vi "Display Lab Panel V4.83.vi"() -> ()   [LabVIEW 2012]
uses:
  Global display 1.vi
  Global display 2.vi
panel:
  in  "Tab Control 2":T1(tab)
  out "SIG LAB05-2":T2 {"PF" format="%.2f"; "AMPS" format="%.1f"}
  out "SIG LAB05-1":T2 {"PF" format="%.2f"; "AMPS" format="%.1f"}
  out "SIG LAB04-2":T2 {"PF" format="%.2f"; "AMPS" format="%.1f"}
  out "SIG LAB04-1":T2 {"PF" format="%.2f"; "AMPS" format="%.1f"}
  out "SIG LAB03-2":T2 {"PF" format="%.2f"; "AMPS" format="%.1f"}
  out "SIG LAB03-1":T2 {"PF" format="%.2f"; "AMPS" format="%.1f"}
  out "SIG LAB02-2":T2 {"PF" format="%.2f"; "AMPS" format="%.1f"}
  in  "RUN LAB01-1":bool
  in  "O/I  LAB05-1":bool
  in  "O/I  LAB05-2":bool
  in  "O/I  LAB04-1":bool
  in  "O/I  LAB04-2":bool
  in  "O/I  LAB02-1":bool
  in  "O/I  LAB02-2":bool
  in  "O/I  LAB01-2":bool
  in  "O/I  LAB01-1":bool
  in  "O/I  LAB03-1":bool
  in  "RUN LAB05-2":bool
  in  "RUN LAB05-1":bool
  in  "RUN LAB04-2":bool
  in  "RUN LAB04-1":bool
  in  "RUN LAB03-2":bool
  in  "RUN LAB03-1":bool
  in  "RUN LAB02-2":bool
  in  "RUN LAB02-1":bool
  in  "RUN LAB01-2":bool
  in  "SELECT LAB05-2":T3(radio)
  in  "SELECT LAB05-1":T3(radio)
  in  "SELECT LAB04-2":T3(radio)
  in  "SELECT LAB04-1":T3(radio)
  in  "SELECT LAB03-2":T3(radio)
  in  "SELECT LAB03-1":T3(radio)
  in  "SELECT LAB02-2":T3(radio)
  in  "SELECT LAB02-1":T3(radio)
  in  "SELECT LAB01-2":T3(radio)
  in  "SELECT LAB01-1":T3(radio)
  in  "O/I  LAB03-2":bool
  out "SIG LAB01-1":T2 {"PF" format="%.2f"; "AMPS" format="%.1f"}
  out "SIG LAB01-2":T2 {"PF" format="%.2f"; "AMPS" format="%.1f"}
  out "SIG LAB02-1":T2 {"PF" format="%.2f"; "AMPS" format="%.1f"}
  out "DISP LAB05-2":T4 {"MINS" format="%.2g"}
  out "DISP LAB05-1":T4 {"MINS" format="%.2g"}
  out "DISP LAB04-2":T4 {"MINS" format="%.2g"}
  out "DISP LAB04-1":T4 {"MINS" format="%.2g"}
  out "DISP LAB03-2":T4 {"MINS" format="%.2g"}
  out "DISP LAB03-1":T4 {"MINS" format="%.2g"}
  in  "SET LAB05-2":T5={"NAME"="", "DESCRIPTION"="", "CYCLES"=5.0, "T-RISE mins"=0.0, "T-RISE deg C"=0.0} {"CYCLES" min=5.0 step=1.0}
  in  "SET LAB05-1":T5={"NAME"="", "DESCRIPTION"="", "CYCLES"=5.0, "T-RISE mins"=0.0, "T-RISE deg C"=0.0} {"CYCLES" min=5.0 step=1.0}
  in  "SET LAB04-2":T5={"NAME"="", "DESCRIPTION"="", "CYCLES"=5.0, "T-RISE mins"=0.0, "T-RISE deg C"=0.0} {"CYCLES" min=5.0 step=1.0}
  in  "SET LAB04-1":T5={"NAME"="", "DESCRIPTION"="", "CYCLES"=5.0, "T-RISE mins"=0.0, "T-RISE deg C"=0.0} {"CYCLES" min=5.0 step=1.0}
  in  "SET LAB03-2":T5={"NAME"="", "DESCRIPTION"="", "CYCLES"=5.0, "T-RISE mins"=0.0, "T-RISE deg C"=0.0} {"CYCLES" min=5.0 step=1.0}
  in  "SET LAB03-1":T5={"NAME"="", "DESCRIPTION"="", "CYCLES"=5.0, "T-RISE mins"=0.0, "T-RISE deg C"=0.0} {"CYCLES" min=5.0 step=1.0}
  out "DISP LAB02-2":T4 {"MINS" format="%.2g"}
  out "DISP LAB02-1":T4 {"MINS" format="%.2g"}
  in  "SET LAB02-2":T5={"NAME"="", "DESCRIPTION"="", "CYCLES"=5.0, "T-RISE mins"=0.0, "T-RISE deg C"=0.0} {"CYCLES" min=5.0 step=1.0}
  in  "SET LAB02-1":T5={"NAME"="", "DESCRIPTION"="", "CYCLES"=5.0, "T-RISE mins"=0.0, "T-RISE deg C"=0.0} {"CYCLES" min=5.0 step=1.0}
  out "RESULT LAB05-2":bool
  out "RESULT LAB05-1":bool
  out "RESULT LAB04-2":bool
  out "RESULT LAB04-1":bool
  out "RESULT LAB03-2":bool
  out "RESULT LAB03-1":bool
  out "RESULT LAB02-2":bool
  out "RESULT LAB02-1":bool
  out "RESULT LAB01-2":bool
  out "RESULT LAB01-1":bool
  in  "SET LAB01-1":T5={"NAME"="", "DESCRIPTION"="", "CYCLES"=5.0, "T-RISE mins"=0.0, "T-RISE deg C"=0.0} {"CYCLES" min=5.0 step=1.0}
  in  "SET LAB01-2":T5={"NAME"="", "DESCRIPTION"="", "CYCLES"=5.0, "T-RISE mins"=0.0, "T-RISE deg C"=0.0} {"CYCLES" min=5.0 step=1.0}
  out "DISP LAB01-1":T4 {"MINS" format="%.2g"}
  out "DISP LAB01-2":T4 {"MINS" format="%.2f"}
  out "TEST VOLTS CHART":dynamicdata(graph)
  out "TEST AMPS CHART":dynamicdata(graph)
  out "TEMPERATURE (N) CHART":dynamicdata(graph)
  out "TEMPERATURE (L) CHART":dynamicdata(graph)
  # "LAB01"
  # "LAB02"
  # "LAB05"
  # "LAB03"
  # "LAB04"
  # "LAB01"
  # "LAB02"
  # "LAB03"
  # "LAB04"
  # "LAB05"
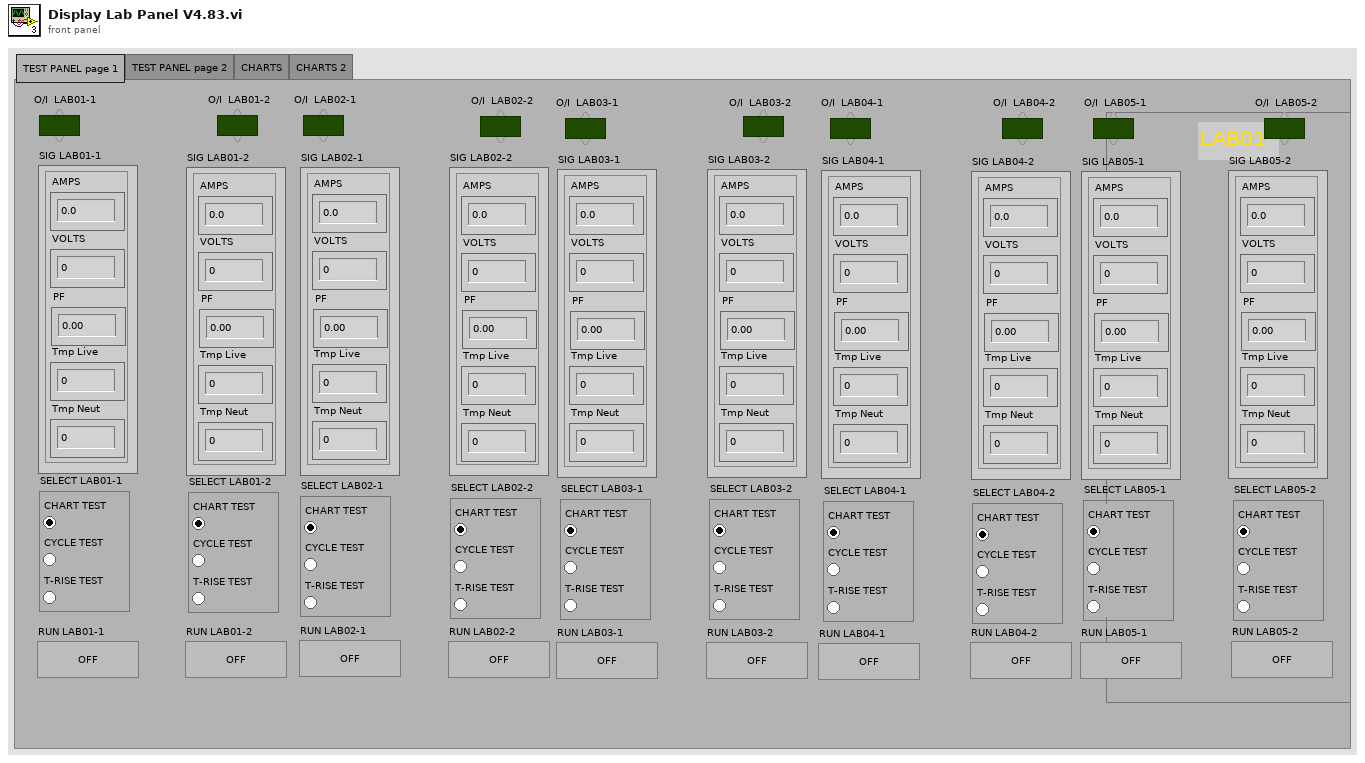
[diagram p1: front panel]
types:
  T1 = enum32{"TEST PANEL page 1", "TEST PANEL page 2", "CHARTS", "CHARTS 2"}
  T2 = cluster{"AMPS":dbl, "VOLTS":dbl, "PF":dbl, "Tmp Live":dbl, "Tmp Neut":dbl}
  T3 = enum32{"CHART TEST", "CYCLE TEST", "T-RISE TEST"}
  T4 = cluster{"CYCLE":dbl, "MINS":dbl, "STATUS":string}
  T5 = cluster{"NAME":string, "DESCRIPTION":string, "CYCLES":dbl, "T-RISE mins":dbl, "T-RISE deg C":dbl}
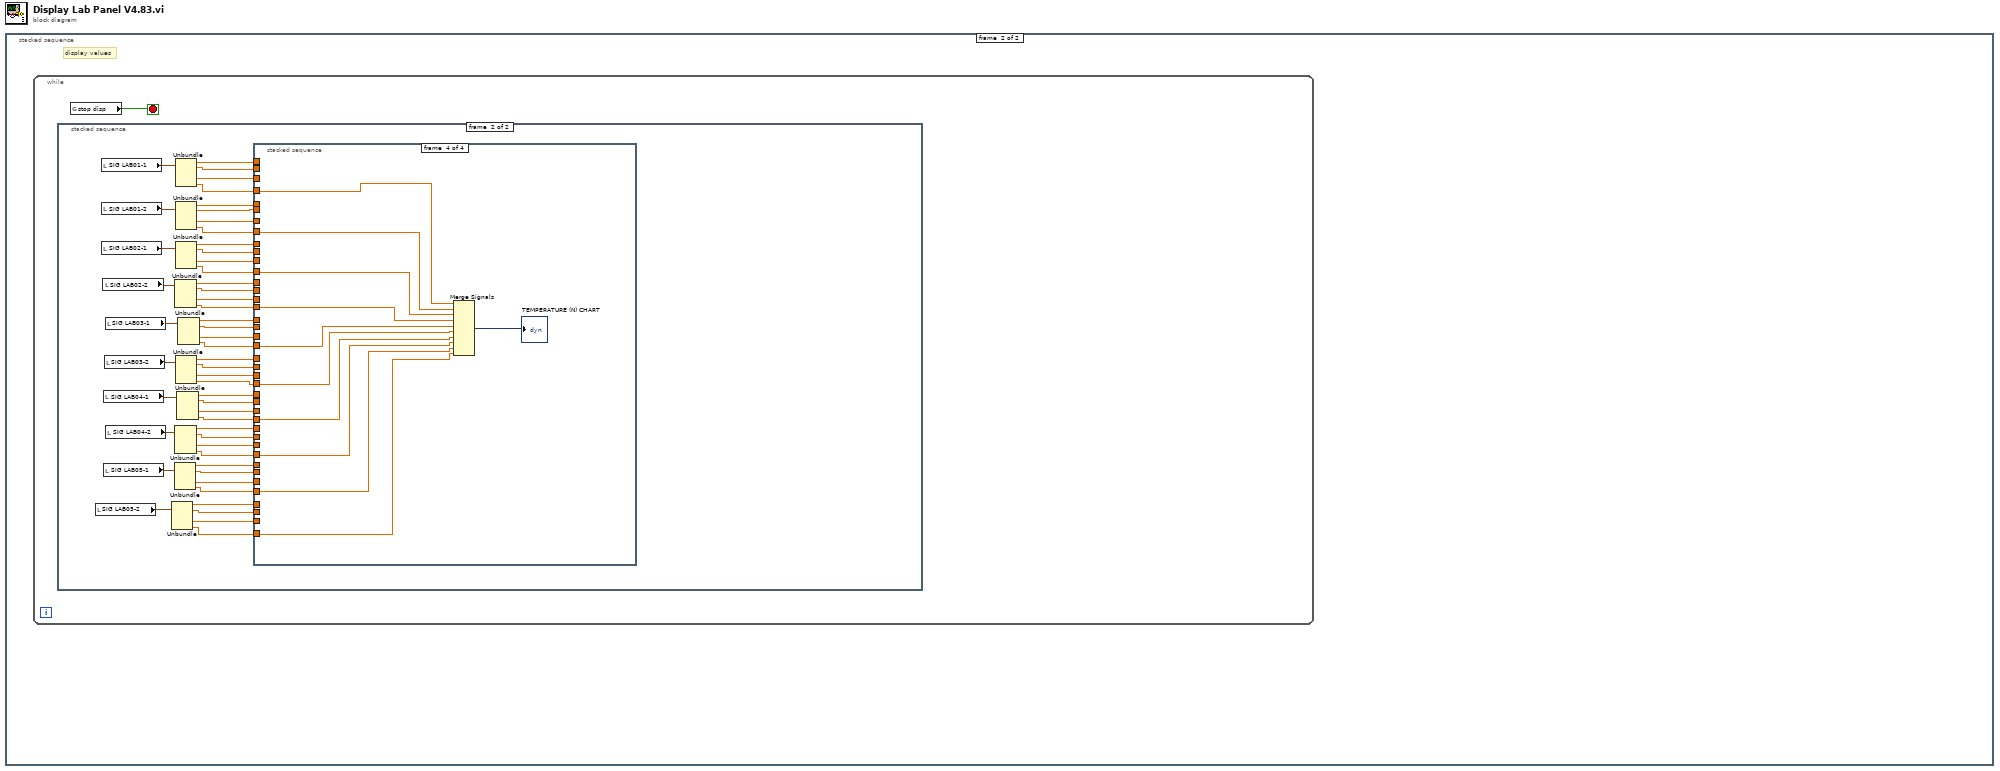
[diagram p0: block diagram]
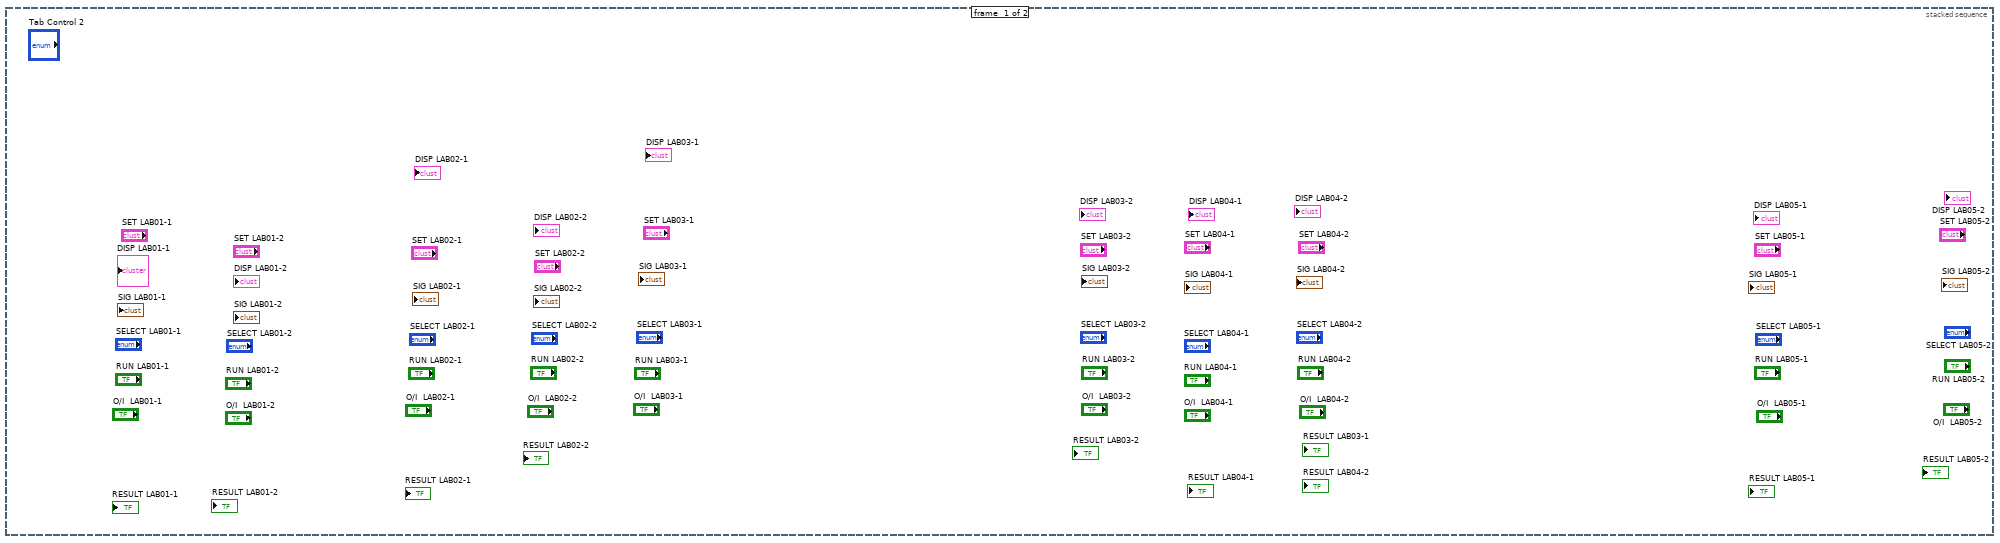
[diagram p2: hidden frame]
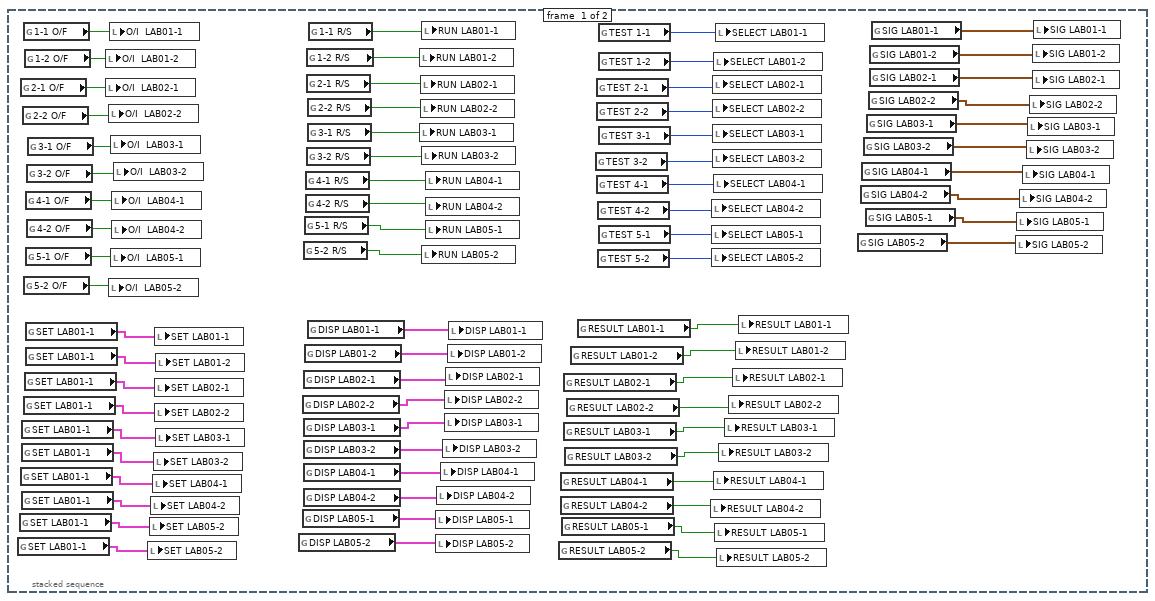
[diagram p3: hidden frame]
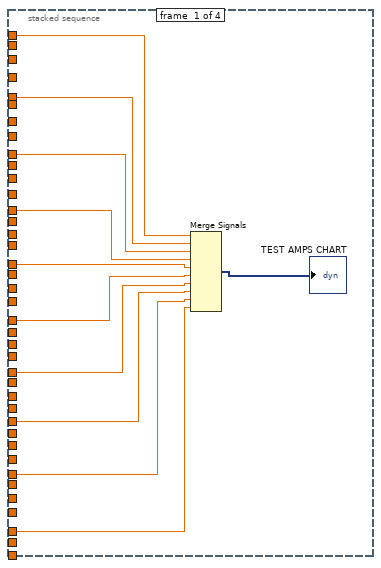
[diagram p4: hidden frame]
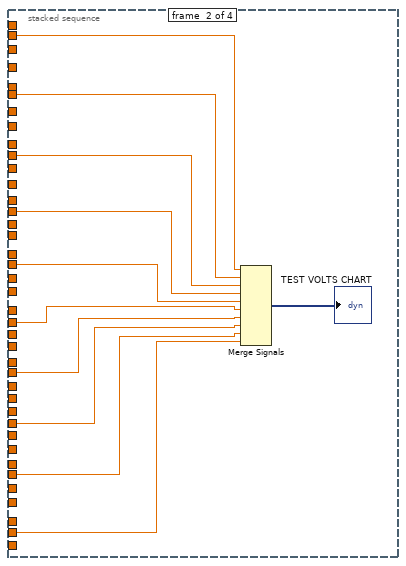
[diagram p5: hidden frame]
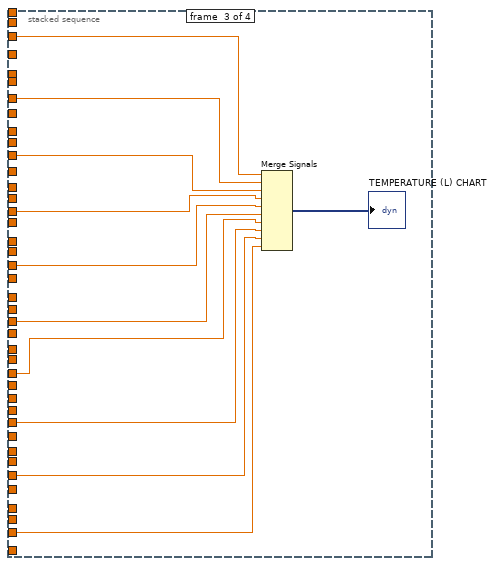
[diagram p6: hidden frame]
diagram:
  n1 = stacked-sequence {
    frame #0 {
    }
    frame #1 {
      # "display values"
      n2 = while {
        stop <- w1 stop-if-true
        n3 = stacked-sequence {
          frame #0 {
            n4 = global read "Global display 2.vi" "SET LAB01-1"() -> (w22:T5)
            n5 = global read "Global display 2.vi" "SET LAB01-1"() -> (w23:T5)
            n6 = global read "Global display 1.vi" "2-1 O/F"() -> (w69:bool)
            n7 = global read "Global display 2.vi" "SET LAB01-1"() -> (w25:T5)
            n8 = global read "Global display 2.vi" "SET LAB01-1"() -> (w27:T5)
            n9 = global read "Global display 2.vi" "SET LAB01-1"() -> (w26:T5)
            n10 = global read "Global display 2.vi" "SET LAB01-1"() -> (w24:T5)
            n11 = global read "Global display 1.vi" "2-2 O/F"() -> (w68:bool)
            n12 = global read "Global display 1.vi" "1-1 O/F"() -> (w71:bool)
            n13 = global read "Global display 1.vi" "5-2 O/F"() -> (w62:bool)
            n14 = global read "Global display 2.vi" "SET LAB01-1"() -> (w28:T5)
            n15 = global read "Global display 1.vi" "1-2 O/F"() -> (w70:bool)
            n16 = global read "Global display 2.vi" "SET LAB01-1"() -> (w29:T5)
            n17 = global read "Global display 1.vi" "4-1 O/F"() -> (w65:bool)
            n18 = global read "Global display 1.vi" "5-1 O/F"() -> (w63:bool)
            n19 = global read "Global display 2.vi" "SET LAB01-1"() -> (w31:T5)
            n20 = global read "Global display 2.vi" "SET LAB01-1"() -> (w30:T5)
            n21 = global read "Global display 1.vi" "3-2 O/F"() -> (w66:bool)
            n22 = global read "Global display 1.vi" "4-2 O/F"() -> (w64:bool)
            n23 = global read "Global display 1.vi" "3-1 O/F"() -> (w67:bool)
            n24 = local write "O/I  LAB01-2"(w70) -> ()
            n25 = local write "O/I  LAB02-1"(w69) -> ()
            n26 = local write "O/I  LAB02-2"(w68) -> ()
            n27 = local write "O/I  LAB05-2"(w62) -> ()
            n28 = local write "O/I  LAB01-1"(w71) -> ()
            n29 = local write "O/I  LAB03-1"(w67) -> ()
            n30 = local write "O/I  LAB05-1"(w63) -> ()
            n31 = local write "O/I  LAB04-1"(w65) -> ()
            n32 = local write "O/I  LAB04-2"(w64) -> ()
            n33 = local write "O/I  LAB03-2"(w66) -> ()
            n34 = local write "SET LAB05-2"(w22) -> ()
            n35 = local write "SET LAB05-2"(w23) -> ()
            n36 = local write "SET LAB04-2"(w24) -> ()
            n37 = local write "SET LAB04-1"(w25) -> ()
            n38 = local write "SET LAB03-2"(w26) -> ()
            n39 = local write "SET LAB01-1"(w31) -> ()
            n40 = local write "SET LAB02-1"(w29) -> ()
            n41 = local write "SET LAB02-2"(w28) -> ()
            n42 = local write "SET LAB01-2"(w30) -> ()
            n43 = local write "SET LAB03-1"(w27) -> ()
            n44 = global read "Global display 2.vi" "DISP LAB05-2"() -> (w12:T4)
            n45 = global read "Global display 2.vi" "DISP LAB02-2"() -> (w18:T4)
            n46 = global read "Global display 2.vi" "DISP LAB05-1"() -> (w13:T4)
            n47 = global read "Global display 1.vi" "5-2 R/S"() -> (w52:bool)
            n48 = global read "Global display 2.vi" "DISP LAB02-1"() -> (w19:T4)
            n49 = global read "Global display 2.vi" "DISP LAB03-1"() -> (w17:T4)
            n50 = global read "Global display 2.vi" "DISP LAB03-2"() -> (w16:T4)
            n51 = global read "Global display 2.vi" "DISP LAB04-1"() -> (w15:T4)
            n52 = global read "Global display 2.vi" "DISP LAB04-2"() -> (w14:T4)
            n53 = global read "Global display 1.vi" "5-1 R/S"() -> (w53:bool)
            n54 = global read "Global display 2.vi" "DISP LAB01-2"() -> (w20:T4)
            n55 = global read "Global display 1.vi" "4-1 R/S"() -> (w55:bool)
            n56 = global read "Global display 1.vi" "4-2 R/S"() -> (w54:bool)
            n57 = global read "Global display 1.vi" "1-2 R/S"() -> (w60:bool)
            n58 = global read "Global display 1.vi" "2-1 R/S"() -> (w59:bool)
            n59 = global read "Global display 1.vi" "3-2 R/S"() -> (w56:bool)
            n60 = global read "Global display 1.vi" "2-2 R/S"() -> (w58:bool)
            n61 = global read "Global display 1.vi" "3-1 R/S"() -> (w57:bool)
            n62 = global read "Global display 2.vi" "DISP LAB01-1"() -> (w21:T4)
            n63 = global read "Global display 1.vi" "1-1 R/S"() -> (w61:bool)
            n64 = local write "RUN LAB01-2"(w60) -> ()
            n65 = local write "RUN LAB03-1"(w57) -> ()
            n66 = local write "RUN LAB02-1"(w59) -> ()
            n67 = local write "RUN LAB02-2"(w58) -> ()
            n68 = local write "RUN LAB01-1"(w61) -> ()
            n69 = local write "RUN LAB03-2"(w56) -> ()
            n70 = local write "RUN LAB05-2"(w52) -> ()
            n71 = local write "RUN LAB04-1"(w55) -> ()
            n72 = local write "RUN LAB04-2"(w54) -> ()
            n73 = local write "RUN LAB05-1"(w53) -> ()
            n74 = local write "DISP LAB05-1"(w13) -> ()
            n75 = local write "DISP LAB05-2"(w12) -> ()
            n76 = local write "DISP LAB04-2"(w14) -> ()
            n77 = local write "DISP LAB04-1"(w15) -> ()
            n78 = local write "DISP LAB03-2"(w16) -> ()
            n79 = local write "DISP LAB02-2"(w18) -> ()
            n80 = local write "DISP LAB03-1"(w17) -> ()
            n81 = local write "DISP LAB02-1"(w19) -> ()
            n82 = local write "DISP LAB01-2"(w20) -> ()
            n83 = local write "DISP LAB01-1"(w21) -> ()
            n84 = global read "Global display 2.vi" "RESULT LAB05-2"() -> (w2:bool)
            n85 = global read "Global display 2.vi" "RESULT LAB04-1"() -> (w5:bool)
            n86 = global read "Global display 2.vi" "RESULT LAB04-2"() -> (w4:bool)
            n87 = global read "Global display 2.vi" "RESULT LAB05-1"() -> (w3:bool)
            n88 = global read "Global display 2.vi" "RESULT LAB02-1"() -> (w9:bool)
            n89 = global read "Global display 2.vi" "RESULT LAB03-1"() -> (w7:bool)
            n90 = global read "Global display 2.vi" "RESULT LAB03-2"() -> (w6:bool)
            n91 = global read "Global display 2.vi" "RESULT LAB02-2"() -> (w8:bool)
            n92 = global read "Global display 2.vi" "RESULT LAB01-2"() -> (w10:bool)
            n93 = global read "Global display 2.vi" "RESULT LAB01-1"() -> (w11:bool)
            n94 = global read "Global display 1.vi" "TEST 3-2"() -> (w46:T3)
            n95 = global read "Global display 1.vi" "TEST 2-1"() -> (w49:T3)
            n96 = global read "Global display 1.vi" "TEST 2-2"() -> (w48:T3)
            n97 = global read "Global display 1.vi" "TEST 4-1"() -> (w45:T3)
            n98 = global read "Global display 1.vi" "TEST 4-2"() -> (w44:T3)
            n99 = global read "Global display 1.vi" "TEST 5-2"() -> (w42:T3)
            n100 = global read "Global display 1.vi" "TEST 1-1"() -> (w51:T3)
            n101 = global read "Global display 1.vi" "TEST 1-2"() -> (w50:T3)
            n102 = global read "Global display 1.vi" "TEST 3-1"() -> (w47:T3)
            n103 = global read "Global display 1.vi" "TEST 5-1"() -> (w43:T3)
            n104 = local write "RESULT LAB04-2"(w4) -> ()
            n105 = local write "SELECT LAB04-2"(w44) -> ()
            n106 = local write "SELECT LAB05-1"(w43) -> ()
            n107 = local write "SELECT LAB05-2"(w42) -> ()
            n108 = local write "SELECT LAB02-1"(w49) -> ()
            n109 = local write "SELECT LAB02-2"(w48) -> ()
            n110 = local write "SELECT LAB03-1"(w47) -> ()
            n111 = local write "SELECT LAB03-2"(w46) -> ()
            n112 = local write "SELECT LAB01-2"(w50) -> ()
            n113 = local write "SELECT LAB04-1"(w45) -> ()
            n114 = local write "RESULT LAB04-1"(w5) -> ()
            n115 = local write "RESULT LAB05-1"(w3) -> ()
            n116 = local write "SELECT LAB01-1"(w51) -> ()
            n117 = local write "RESULT LAB05-2"(w2) -> ()
            n118 = local write "RESULT LAB03-2"(w6) -> ()
            n119 = local write "RESULT LAB03-1"(w7) -> ()
            n120 = local write "RESULT LAB02-2"(w8) -> ()
            n121 = local write "RESULT LAB02-1"(w9) -> ()
            n122 = local write "RESULT LAB01-2"(w10) -> ()
            n123 = local write "RESULT LAB01-1"(w11) -> ()
            n124 = global read "Global display 1.vi" "SIG LAB05-2"() -> (w32:T2)
            n125 = global read "Global display 1.vi" "SIG LAB04-2"() -> (w34:T2)
            n126 = global read "Global display 1.vi" "SIG LAB04-1"() -> (w35:T2)
            n127 = global read "Global display 1.vi" "SIG LAB03-2"() -> (w36:T2)
            n128 = global read "Global display 1.vi" "SIG LAB05-1"() -> (w33:T2)
            n129 = global read "Global display 1.vi" "SIG LAB03-1"() -> (w37:T2)
            n130 = global read "Global display 1.vi" "SIG LAB02-2"() -> (w38:T2)
            n131 = global read "Global display 1.vi" "SIG LAB01-2"() -> (w40:T2)
            n132 = global read "Global display 1.vi" "SIG LAB02-1"() -> (w39:T2)
            n133 = global read "Global display 1.vi" "SIG LAB01-1"() -> (w41:T2)
            n134 = local write "SIG LAB05-2"(w32) -> ()
            n135 = local write "SIG LAB05-1"(w33) -> ()
            n136 = local write "SIG LAB04-2"(w34) -> ()
            n137 = local write "SIG LAB04-1"(w35) -> ()
            n138 = local write "SIG LAB03-2"(w36) -> ()
            n139 = local write "SIG LAB03-1"(w37) -> ()
            n140 = local write "SIG LAB02-2"(w38) -> ()
            n141 = local write "SIG LAB01-2"(w40) -> ()
            n142 = local write "SIG LAB02-1"(w39) -> ()
            n143 = local write "SIG LAB01-1"(w41) -> ()
          }
          frame #1 {
            n144 = local read "SIG LAB05-2"() -> (w112:T2)
            n145 = local read "SIG LAB01-1"() -> (w121:T2)
            n146 = local read "SIG LAB01-2"() -> (w120:T2)
            n147 = local read "SIG LAB02-1"() -> (w119:T2)
            n148 = local read "SIG LAB02-2"() -> (w118:T2)
            n149 = local read "SIG LAB04-1"() -> (w115:T2)
            n150 = local read "SIG LAB05-1"() -> (w113:T2)
            n151 = local read "SIG LAB03-2"() -> (w116:T2)
            n152 = local read "SIG LAB03-1"() -> (w117:T2)
            n153 = local read "SIG LAB04-2"() -> (w114:T2)
            n154 = Unbundle(w112) -> ("AMPS"=w102:dbl, "VOLTS"=w92:dbl, "Tmp Live"=w82:dbl, "Tmp Neut"=w72:dbl)  [unwired: 1 out]
            n155 = Unbundle(w113) -> ("AMPS"=w103:dbl, "VOLTS"=w93:dbl, "Tmp Live"=w83:dbl, "Tmp Neut"=w73:dbl)  [unwired: 1 out]
            n156 = Unbundle(w118) -> ("AMPS"=w108:dbl, "VOLTS"=w98:dbl, "Tmp Live"=w88:dbl, "Tmp Neut"=w78:dbl)  [unwired: 1 out]
            n157 = Unbundle(w114) -> ("AMPS"=w104:dbl, "VOLTS"=w94:dbl, "Tmp Live"=w85:dbl, "Tmp Neut"=w74:dbl)  [unwired: 1 out]
            n158 = Unbundle(w121) -> ("AMPS"=w111:dbl, "VOLTS"=w101:dbl, "Tmp Live"=w91:dbl, "Tmp Neut"=w81:dbl)  [unwired: 1 out]
            n159 = Unbundle(w120) -> ("AMPS"=w110:dbl, "VOLTS"=w100:dbl, "Tmp Live"=w90:dbl, "Tmp Neut"=w80:dbl)  [unwired: 1 out]
            n160 = Unbundle(w119) -> ("AMPS"=w109:dbl, "VOLTS"=w99:dbl, "Tmp Live"=w89:dbl, "Tmp Neut"=w79:dbl)  [unwired: 1 out]
            n161 = Unbundle(w116) -> ("AMPS"=w106:dbl, "VOLTS"=w96:dbl, "Tmp Live"=w86:dbl, "Tmp Neut"=w76:dbl)  [unwired: 1 out]
            n162 = Unbundle(w115) -> ("AMPS"=w105:dbl, "VOLTS"=w95:dbl, "Tmp Live"=w84:dbl, "Tmp Neut"=w75:dbl)  [unwired: 1 out]
            n163 = Unbundle(w117) -> ("AMPS"=w107:dbl, "VOLTS"=w97:dbl, "Tmp Live"=w87:dbl, "Tmp Neut"=w77:dbl)  [unwired: 1 out]
            n164 = stacked-sequence {
              tunnel: w111 -> [w132 _ _ _]
              tunnel: w110 -> [w131 _ _ _]
              tunnel: w109 -> [w130 _ _ _]
              tunnel: w108 -> [w129 _ _ _]
              tunnel: w107 -> [w128 _ _ _]
              tunnel: w106 -> [w127 _ _ _]
              tunnel: w105 -> [w126 _ _ _]
              tunnel: w104 -> [w125 _ _ _]
              tunnel: w103 -> [w124 _ _ _]
              tunnel: w102 -> [w123 _ _ _]
              tunnel: w101 -> [_ w143 _ _]
              tunnel: w100 -> [_ w142 _ _]
              tunnel: w99 -> [_ w141 _ _]
              tunnel: w98 -> [_ w140 _ _]
              tunnel: w97 -> [_ w139 _ _]
              tunnel: w96 -> [_ w138 _ _]
              tunnel: w95 -> [_ w137 _ _]
              tunnel: w94 -> [_ w136 _ _]
              tunnel: w93 -> [_ w135 _ _]
              tunnel: w92 -> [_ w134 _ _]
              tunnel: w91 -> [_ _ w154 _]
              tunnel: w90 -> [_ _ w153 _]
              tunnel: w89 -> [_ _ w152 _]
              tunnel: w88 -> [_ _ w151 _]
              tunnel: w87 -> [_ _ w150 _]
              tunnel: w86 -> [_ _ w149 _]
              tunnel: w85 -> [_ _ w147 _]
              tunnel: w84 -> [_ _ w148 _]
              tunnel: w83 -> [_ _ w146 _]
              tunnel: w82 -> [_ _ w145 _]
              tunnel: w81 -> [_ _ _ w165]
              tunnel: w80 -> [_ _ _ w164]
              tunnel: w79 -> [_ _ _ w163]
              tunnel: w78 -> [_ _ _ w162]
              tunnel: w77 -> [_ _ _ w161]
              tunnel: w76 -> [_ _ _ w160]
              tunnel: w75 -> [_ _ _ w159]
              tunnel: w74 -> [_ _ _ w158]
              tunnel: w73 -> [_ _ _ w157]
              tunnel: w72 -> [_ _ _ w156]
              frame #0 {
                n165 = Merge Signals(w132, w131, w130, w129, w128, w127, w126, w125, w124, w123) -> (→"TEST AMPS CHART":dynamicdata)
              }
              frame #1 {
                n166 = Merge Signals(w143, w142, w141, w140, w139, w138, w137, w136, w135, w134) -> (→"TEST VOLTS CHART":dynamicdata)
              }
              frame #2 {
                n167 = Merge Signals(w154, w153, w152, w151, w150, w149, w148, w147, w146, w145) -> (→"TEMPERATURE (L) CHART":dynamicdata)
              }
              frame #3 {
                n168 = Merge Signals(w165, w164, w163, w162, w161, w160, w159, w158, w157, w156) -> (→"TEMPERATURE (N) CHART":dynamicdata)
              }
            }
          }
        }
        n169 = global read "Global display 1.vi" "stop disp"() -> (w1:bool)
      }
    }
  }
